vi "pf32_spad_array.vi"() -> ()   [LabVIEW 2021]
panel:
  in  "Scanning Type":dbl
  in  "galvo type":i32=1
  out "exposure time":dbl
  out "Index":dbl
  # "1. Around four veritces\n2. All pixels\n3. NLOS Measurement"
  # "1. SEM103不知道哪台笔记本\n2. 1B405慢的电脑\n3. 1B405快的电脑"
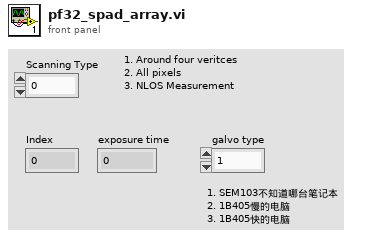
[diagram p1: front panel]
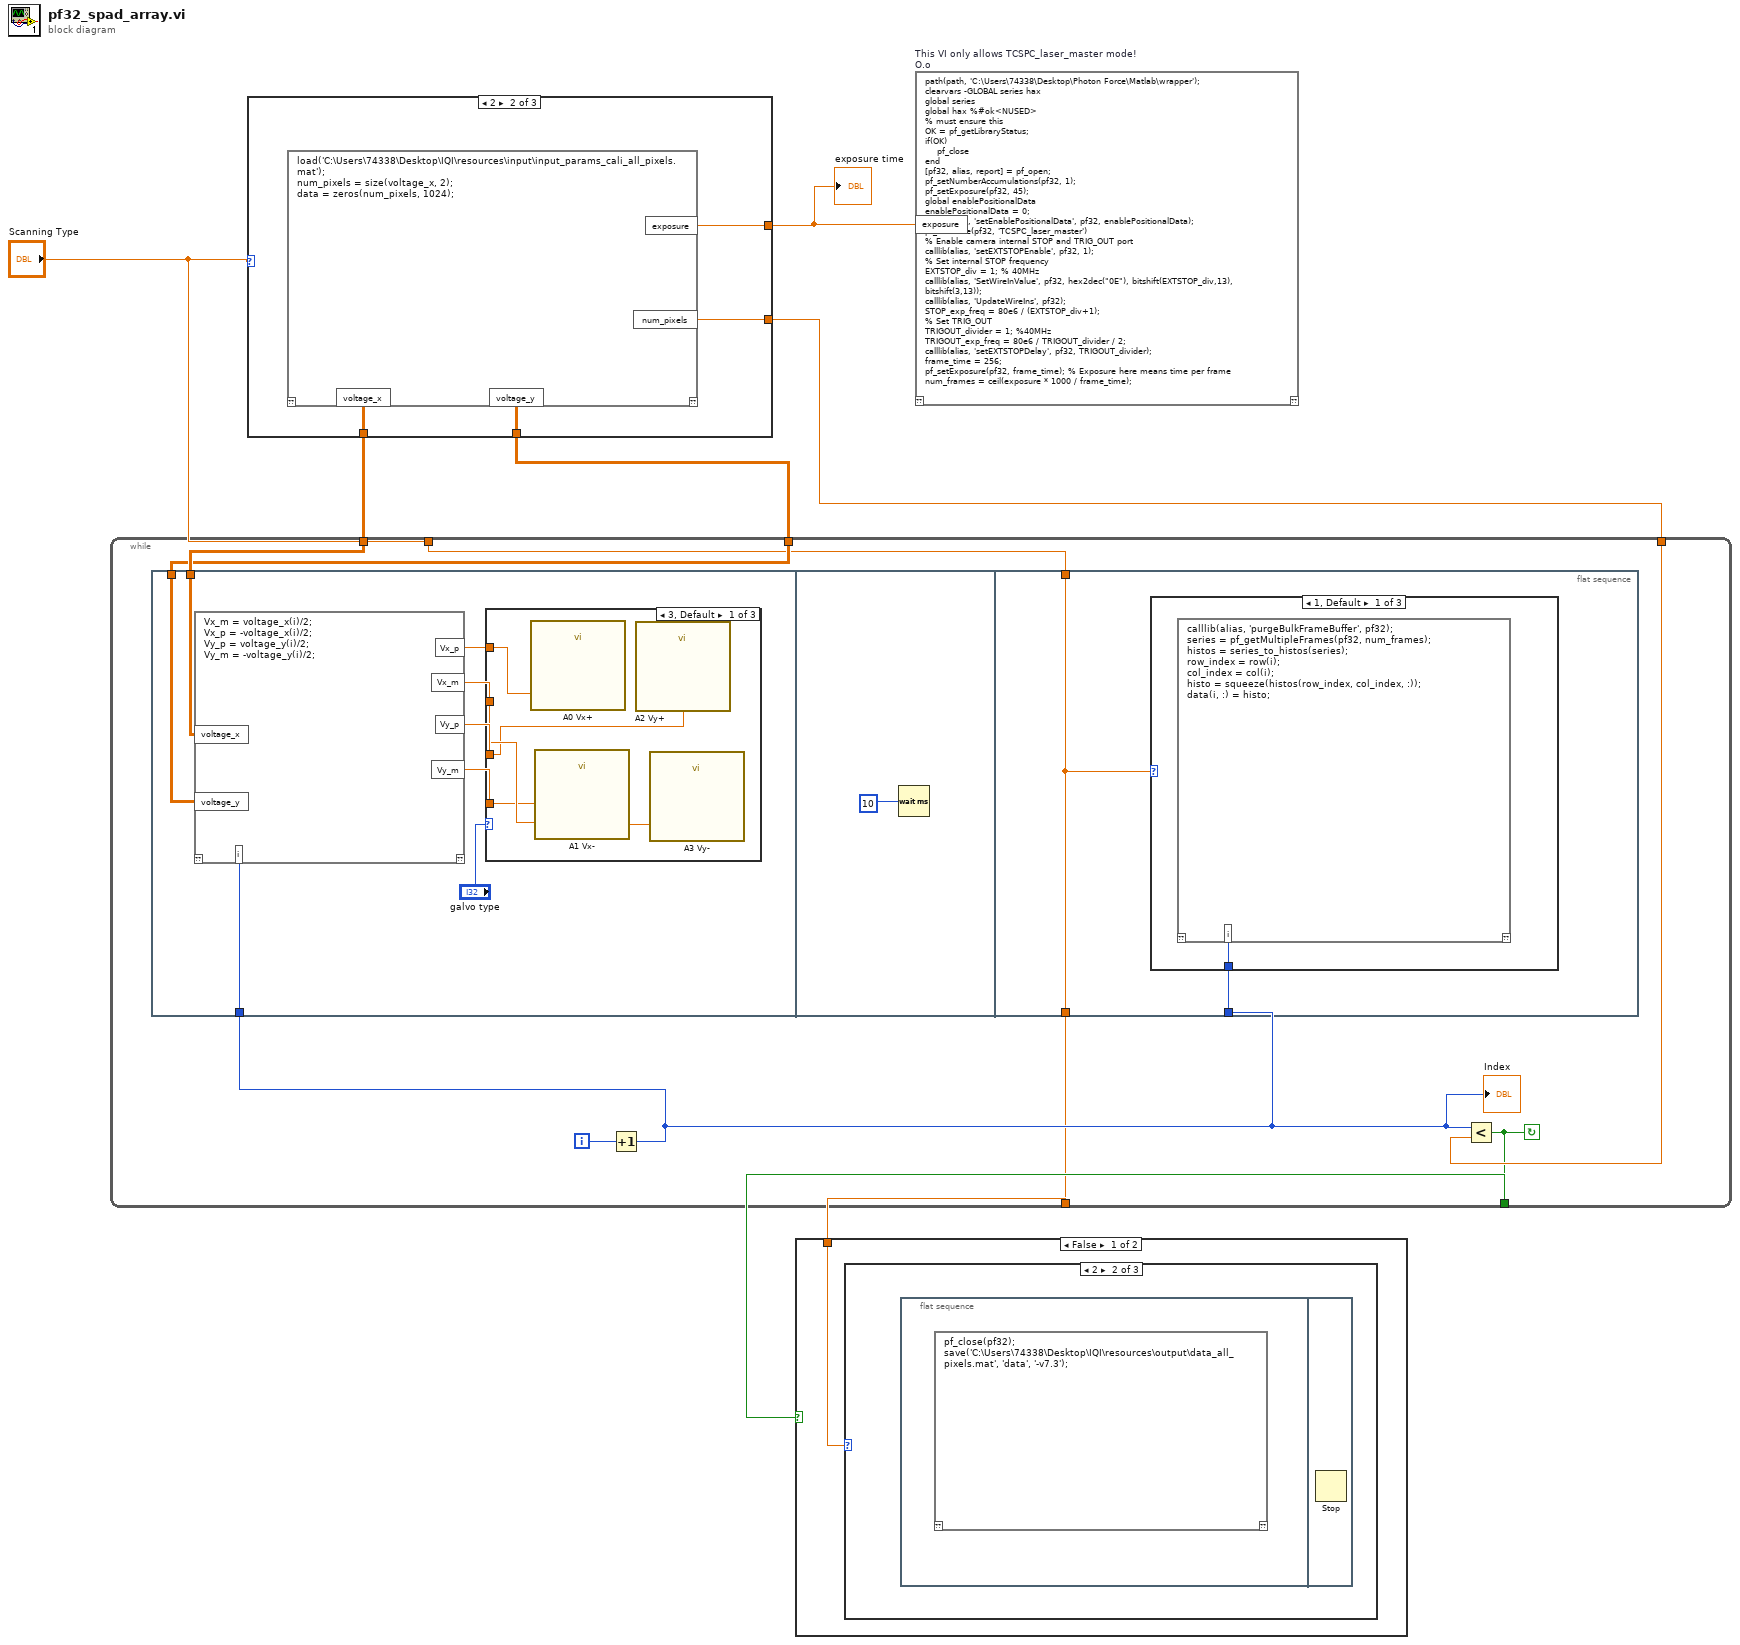
[diagram p0: block diagram]
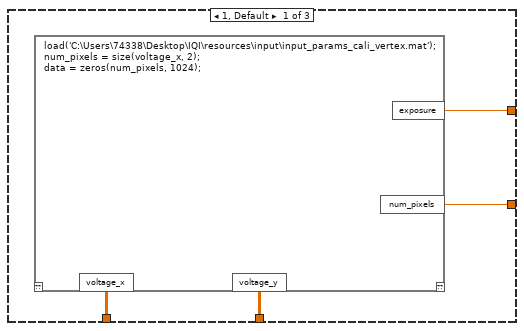
[diagram p2: hidden frame]
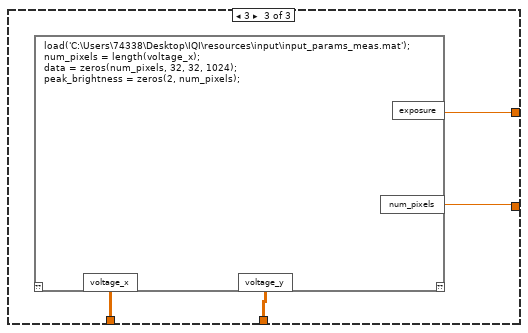
[diagram p3: hidden frame]
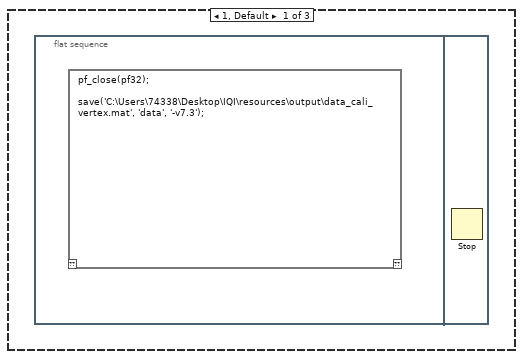
[diagram p4: hidden frame]
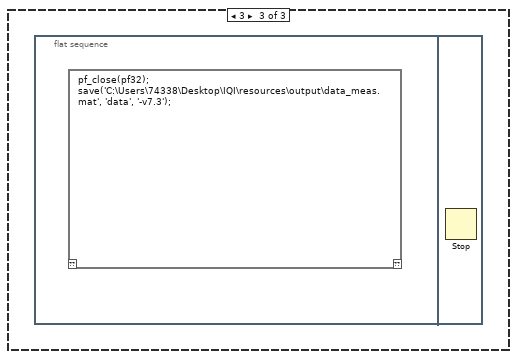
[diagram p5: hidden frame]
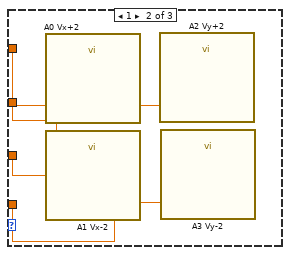
[diagram p7: hidden frame]
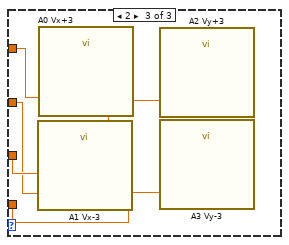
[diagram p8: hidden frame]
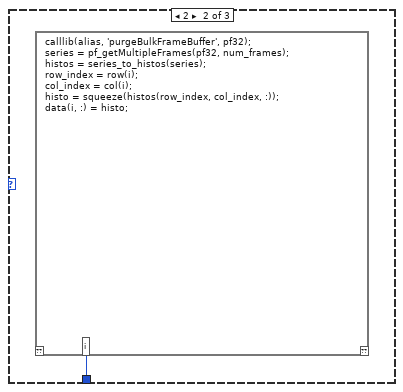
[diagram p9: hidden frame]
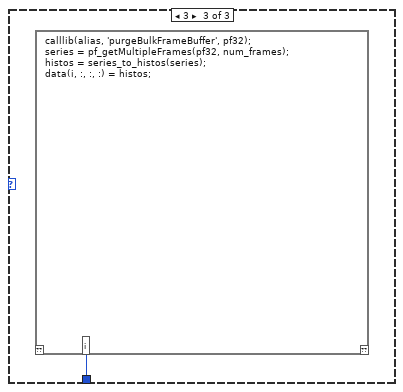
[diagram p10: hidden frame]
diagram:
  n1 = case shown="2" "Scanning Type" {
    tunnel: [w11 w15 w16] -> w7
    tunnel: [w10 w14 w17] -> w6
    tunnel: [w9 w13 w19] -> w5
    tunnel: [w8 w12 w18] -> w4
    frame 1, Default {
      n2 = script code="load('C:\\Users\\74338\\Desktop\\IQI\\resources\\input\\input_params_cali_vertex.mat');\nnum_pixels = size(voltage_x, 2);\ndata = zeros(num_pixels, 1024);"() -> ("voltage_y"=w10:dbl[][], "voltage_x"=w11:dbl[][], "exposure"=w9:dbl, "num_pixels"=w8:dbl)  [unwired: 1 in, 1 out]
    }
    frame 2 {
      n3 = script code="load('C:\\Users\\74338\\Desktop\\IQI\\resources\\input\\input_params_cali_all_pixels.mat');\nnum_pixels = size(voltage_x, 2);\ndata = zeros(num_pixels, 1024);"() -> ("voltage_y"=w14:dbl[][], "voltage_x"=w15:dbl[][], "exposure"=w13:dbl, "num_pixels"=w12:dbl)  [unwired: 1 in, 1 out]
    }
    frame 3 {
      n4 = script code="load('C:\\Users\\74338\\Desktop\\IQI\\resources\\input\\input_params_meas.mat');\nnum_pixels = length(voltage_x);\ndata = zeros(num_pixels, 32, 32, 1024);\npeak_brightness = zeros(2, num_pixels);"() -> ("voltage_y"=w17:dbl[][], "voltage_x"=w16:dbl[][], "exposure"=w19:dbl, "num_pixels"=w18:dbl)  [unwired: 1 in, 1 out]
    }
  }
  "exposure time" <- w5
  n5 = while {
    tunnel: w7 -> [w27]
    tunnel: w6 -> [w26]
    tunnel: w4 -> [w25]
    tunnel: [w24] -> w3
    tunnel: "Scanning Type" -> [w21]
    tunnel: [w20] -> w1
    i -> [w23]
    stop <- w24 continue-if-true
    n6 = flat-sequence {
      tunnel: w27 -> [w30]
      tunnel: w26 -> [w29]
      tunnel: w22 -> [w28]
      tunnel: w22 -> [w50]
      tunnel: w21 -> [w49]
      tunnel: [w49] -> w20
      frame #0 {
        n7 = script code="Vx_m = voltage_x(i)/2;\nVx_p = -voltage_x(i)/2;\nVy_p = voltage_y(i)/2;\nVy_m = -voltage_y(i)/2;"("voltage_x"=w30, "i"=w28, "voltage_y"=w29) -> ("Vx_p"=w33:dbl, "Vx_m"=w35:dbl, "Vy_p"=w34:dbl, "Vy_m"=w32:dbl)  [unwired: 1 in, 1 out]
        n8 = case shown="3, Default" "galvo type" {
          tunnel: w35 -> [w39 w43 w44]
          tunnel: w34 -> [w36 w42 w47]
          tunnel: w32 -> [w38 w41 w46]
          tunnel: w33 -> [w37 w40 w45]
          frame 3, Default {
            n9 = call "A0 Vx+"("data"=w37) -> ()  [unwired: 17 in, 2 out]
            n10 = call "A1 Vx-"("data"=w39) -> ()  [unwired: 17 in, 2 out]
            n11 = call "A2 Vy+"("data"=w36) -> ()  [unwired: 17 in, 2 out]
            n12 = call "A3 Vy-"("data"=w38) -> ()  [unwired: 17 in, 2 out]
          }
          frame 1 {
            n13 = call "A0 Vx+2"("data"=w40) -> ()  [unwired: 17 in, 2 out]
            n14 = call "A1 Vx-2"("data"=w43) -> ()  [unwired: 17 in, 2 out]
            n15 = call "A2 Vy+2"("data"=w42) -> ()  [unwired: 17 in, 2 out]
            n16 = call "A3 Vy-2"("data"=w41) -> ()  [unwired: 17 in, 2 out]
          }
          frame 2 {
            n17 = call "A1 Vx-3"("data"=w44) -> ()  [unwired: 17 in, 2 out]
            n18 = call "A0 Vx+3"("data"=w45) -> ()  [unwired: 17 in, 2 out]
            n19 = call "A2 Vy+3"("data"=w47) -> ()  [unwired: 17 in, 2 out]
            n20 = call "A3 Vy-3"("data"=w46) -> ()  [unwired: 17 in, 2 out]
          }
        }
      }
      frame #1 {
        n21 = Wait (ms)(milliseconds to wait=10) -> ()  [unwired: 1 out]
      }
      frame #2 {
        n22 = case shown="1, Default" w49 {
          tunnel: w50 -> [w51 w52 w53]
          frame 1, Default {
            n23 = script code="calllib(alias, 'purgeBulkFrameBuffer', pf32);\nseries = pf_getMultipleFrames(pf32, num_frames);\nhistos = series_to_histos(series);\nrow_index = row(i);\ncol_index = col(i);\nhisto = squeeze(histos(row_index, col_index, :));\ndata(i, :) = histo;"("i"=w51) -> ()  [unwired: 1 in, 1 out]
          }
          frame 2 {
            n24 = script code="calllib(alias, 'purgeBulkFrameBuffer', pf32);\nseries = pf_getMultipleFrames(pf32, num_frames);\nhistos = series_to_histos(series);\nrow_index = row(i);\ncol_index = col(i);\nhisto = squeeze(histos(row_index, col_index, :));\ndata(i, :) = histo;"("i"=w52) -> ()  [unwired: 1 in, 1 out]
          }
          frame 3 {
            n25 = script code="calllib(alias, 'purgeBulkFrameBuffer', pf32);\nseries = pf_getMultipleFrames(pf32, num_frames);\nhistos = series_to_histos(series);\ndata(i, :, :, :) = histos;"("i"=w53) -> ()  [unwired: 1 in, 1 out]
          }
        }
      }
    }
    n26 = Increment(x=w23) -> (x+1=w22:i32)
    "Index" <- w22
    n27 = Less?(x=w22, y=w25) -> (x < y?=w24:bool)
  }
  n28 = case shown="False" w3 {
    tunnel: w1 -> [w54 _]
    frame False {
      n29 = case shown="2" w54 {
        frame 1, Default {
          n30 = flat-sequence {
            frame #0 {
              n31 = script code="pf_close(pf32);\n\nsave('C:\\Users\\74338\\Desktop\\IQI\\resources\\output\\data_cali_vertex.mat', 'data', '-v7.3');"() -> ()  [unwired: 1 in, 1 out]
            }
            frame #1 {
              n32 = Stop() -> ()  [unwired: 1 in]
            }
          }
        }
        frame 2 {
          n33 = flat-sequence {
            frame #0 {
              n34 = script code="pf_close(pf32);\nsave('C:\\Users\\74338\\Desktop\\IQI\\resources\\output\\data_all_pixels.mat', 'data', '-v7.3');"() -> ()  [unwired: 1 in, 1 out]
            }
            frame #1 {
              n35 = Stop() -> ()  [unwired: 1 in]
            }
          }
        }
        frame 3 {
          n36 = flat-sequence {
            frame #0 {
              n37 = script code="pf_close(pf32);\nsave('C:\\Users\\74338\\Desktop\\IQI\\resources\\output\\data_meas.mat', 'data', '-v7.3');"() -> ()  [unwired: 1 in, 1 out]
            }
            frame #1 {
              n38 = Stop() -> ()  [unwired: 1 in]
            }
          }
        }
      }
    }
    frame True {
    }
  }
  n39 = script code="path(path, 'C:\\Users\\74338\\Desktop\\Photon Force\\Matlab\\wrapper');\nclearvars -GLOBAL series hax\nglobal series\nglobal hax %#ok<NUSED>\n% must ensure this\nOK = pf_getLibraryStatus;\nif(OK)\n    pf_close\nend\n[pf32, alias, report] = pf_open;\npf_setNumberAccumulations(pf32, 1);\npf_setExposure(pf32, 45);\nglobal enablePositionalData\nenablePositionalData = 0;\ncalllib(alias, 'setEnablePositionalData', pf32, enablePositionalData);\npf_setMode(pf32, 'TCSPC_laser_master')\n% Enable camera internal STOP and TRIG_OUT port\ncalllib(alias, 'setEXTSTOPEnable', pf32, 1); \n% Set internal STOP frequency\nEXTSTOP_div = 1; % 40MHz \ncalllib(alias, 'SetWireInValue', pf32, hex2dec(\"0E\"), bitshift(EXTSTOP_div,13), bitshift(3,13));\ncalllib(alias, 'UpdateWireIns', pf32);\nSTOP_exp_freq = 80e6 / (EXTSTOP_div+1);\n% Set TRIG_OUT\nTRIGOUT_divider = 1; %40MHz\nTRIGOUT_exp_freq = 80e6 / TRIGOUT_divider / 2;\ncalllib(alias, 'setEXTSTOPDelay', pf32, TRIGOUT_divider);\nframe_time = 256;\npf_setExposure(pf32, frame_time); % Exposure here means time per frame\nnum_frames = ceil(exposure * 1000 / frame_time);" "This VI only allows TCSPC_laser_master mode! O.o"("exposure"=w5) -> ()  [unwired: 1 in, 1 out]
